vi "edit parameters.vi"(8 "error in (no error)":errorcluster, 11 "Task in":refnum<class "Task.lvclass">) -> (0 "error out":errorcluster, 3 "Task out":refnum<class "Task.lvclass">)   [LabVIEW 2020, in "Tasks.lvlib" / "Task.lvclass"]
uses:
  Task.lvclass
  parameters.ctl
panel:
  in  "parameters":T1
  out "Task summary":string
  out "Task Description":string
  in  "Cancel":bool
  in  "Accept":bool
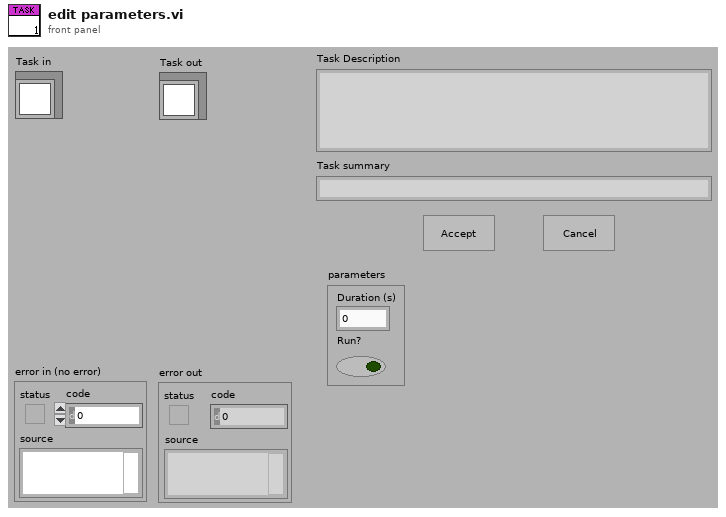
[diagram p1: front panel]
types:
  T1 = typedef "Tasks.lvlib/Task.lvclass/parameters.ctl" = cluster{"Duration (s)":dbl, "Run?":bool}
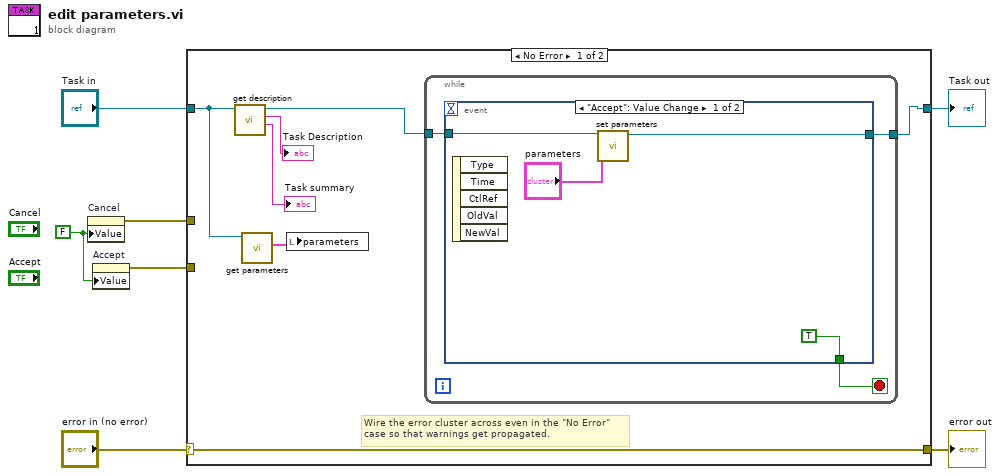
[diagram p0: block diagram]
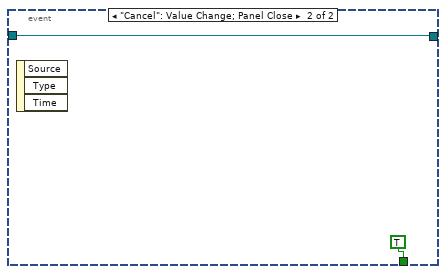
[diagram p2: hidden frame]
diagram:
  w3 = FALSE ("Cancel")
  n1 = property on="Cancel" class="Bool (strict)"("Value"=w3) -> (error out=w2:errorcluster)  [unwired: 2 in, 1 out]
  n2 = property on="Accept" class="Bool (strict)"("Value"=w3) -> (error out=w1:errorcluster)  [unwired: 2 in, 1 out]
  n3 = case shown="No Error" "error in (no error)" {
    selector: "error in (no error)" -> [w14 w25]
    tunnel: [w14 w25] -> w6
    tunnel: [w10 w24] -> w4
    tunnel: "Task in" -> [w9 w24]
    tunnel: w2 -> [_ _]
    tunnel: w1 -> [_ _]
    frame No Error {
      # "Wire the error cluster across even in the \"No Error\"\ncase so that warnings get propagated."
      n4 = call-dynamic "get description.vi"("Task in"=w9) -> ("Task summary"=→"Task summary":string, "Task description"=→"Task Description":string, "Task out"=w11:refnum<class "Task.lvclass">)  [unwired: 7 in, 1 out]
      n5 = call-dynamic "get parameters.vi"("Task.lvclass in"=w9) -> ("parameters"=w8:T1)  [unwired: 8 in, 2 out]
      n6 = local write "parameters"(w8) -> ()
      n7 = while {
        tunnel: w11 -> [w17]
        tunnel: [w16] -> w10
        stop <- w15 stop-if-true
        n8 = event shown="[0] \"Accept\": Value Change" {
          selector: _ -> [_ _]
          dyn-events: _ -> [_ _]
          timeout: _ -> [_ _]
          tunnel: w17 -> [w21 w22]
          tunnel: [w20 w22] -> w16
          tunnel: [TRUE ("NewVal") TRUE ("NewVal")] -> w15
          event "Accept": Value Change {
            n9 = event-data() -> ()  [unwired: 1 in, 5 out]
            n10 = call-dynamic "set parameters.vi"("parameters"="parameters", "Task.lvclass in"=w21) -> ("Task.lvclass out"=w20:refnum<class "Task.lvclass">)  [unwired: 8 in, 1 out]
          }
          event "Cancel": Value Change; Panel Close {
            n11 = event-data() -> ()  [unwired: 1 in, 3 out]
          }
        }
      }
    }
    frame Error {
    }
  }
  "error out" <- w6
  "Task out" <- w4
